vi "GUI Init - DOM6.vi"(7 "Disabled":T1(ring), 8 "error in (no error)":errorcluster, 9 "Ch.names":string[](array[string]), 10 "Cluster":T3, 11 "GUI Refs":T2) -> (0 "error out":errorcluster, 2 "Data":dbl[](array[numeric]), 3 "reference out":refnum<vi>)   [LabVIEW 2017]
doc: "Initialize array's size and values for DOM6 Array by reference"
uses:
  Controls/Discrete_GUI_Cluster.ctl
  Controls/GUI Referencies.ctl
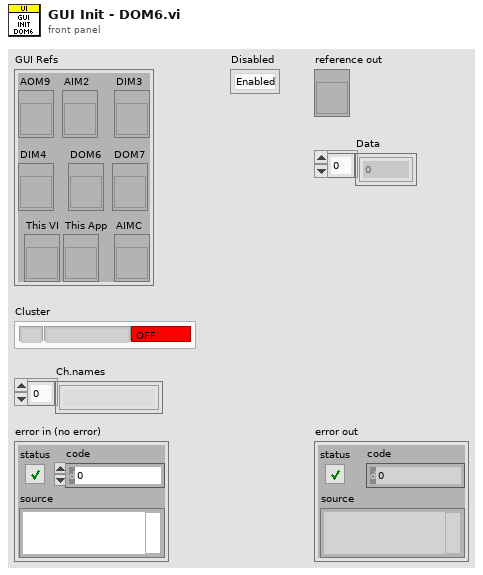
[diagram p1: front panel]
types:
  T1 = enum8{"Enabled", "Disabled", "Disabled and Grayed Out"}
  T2 = typedef "GUI Referencies.ctl" = cluster{"This VI":refnum<vi>, "This App":refnum<vi>, "DIM3":refnum<vi>, "DIM4":refnum<vi>, "DOM6":refnum<vi>, "DOM7":refnum<vi>, "AOM9":refnum<vi>, "AIM2":refnum<vi>, "AIMC":refnum<vi>}
  T3 = typedef "Discrete_GUI_Cluster.ctl" = cluster{"Ch.name":string, "Ch.state":bool, "Num":string}
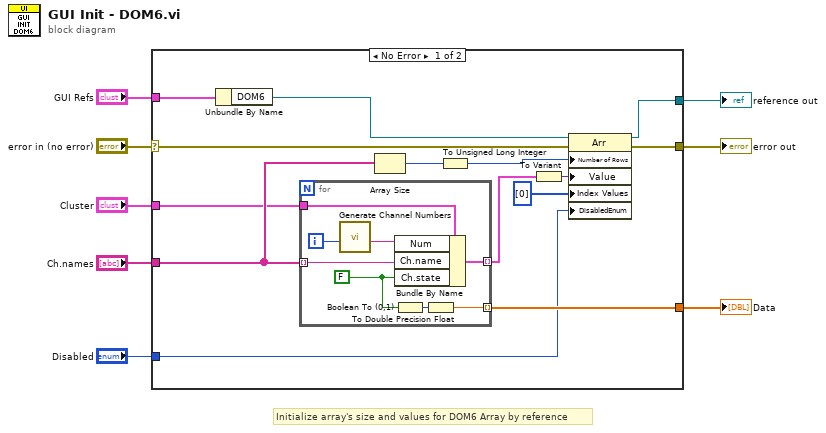
[diagram p0: block diagram]
diagram:
  # "Initialize array's size and values for DOM6 Array by reference"
  n1 = case shown="No Error" "error in (no error)" {
    selector: "error in (no error)" -> [w16 w31]
    tunnel: [w15 w31] -> w7
    tunnel: "Ch.names" -> [w19 _]
    tunnel: "GUI Refs" -> [w18 _]
    tunnel: "Cluster" -> [w17 _]
    tunnel: [w14 _] -> w4
    tunnel: [w10 _] -> w2
    tunnel: "Disabled" -> [w9 _]
    frame No Error {
      n2 = Unbundle By Name(w18) -> ("DOM6"=w11:refnum<vi>)
      n3 = for {
        tunnel: [w30] -> w13 mode=indexing
        tunnel: w19 -> [w29] mode=indexing
        tunnel: w17 -> [w28]
        tunnel: [w25] -> w14 mode=indexing
        i -> [w23]
        w26 = FALSE
        n4 = call "Generate Channel Numbers.vi"("Index"=w23) -> ("Number"=w24:string)  [unwired: 9 in, 1 out]
        n5 = Bundle By Name(cluster=w28, "Num"=w24, "Ch.name"=w29, "Ch.state"=w26) -> (w30:T3)
        n6 = Boolean To (0,1)(Boolean=w26) -> (0, 1=w27:i16)
        n7 = To Double Precision Float(number=w27) -> (double precision float=w25:dbl)
      }
      n8 = Array Size(array=w19) -> (size(s)=w21:i32)
      n9 = To Unsigned Long Integer(number=w21) -> (unsigned 32bit integer=w20:u32)
      n10 = To Variant(anything=w13) -> (Variant=w12:variant)
      n11 = property class="Arr"(reference=w11, error in=w16, "Number of Rows"=w20, "Value"=w12, "Index Values"=u32[] [0], "DisabledEnum"=w9) -> (reference out=w10:refnum<vi>, error out=w15:errorcluster)
    }
    frame Error {
    }
  }
  "error out" <- w7
  "Data" <- w4
  "reference out" <- w2
